vi "Initialize Engine.vi"(8 "error in (no error)":errorcluster, 11 "Abstract Engine":refnum<class "Abstract Engine.lvclass">) -> (0 "error out":errorcluster, 2 "Engine Data":string[](array[string]), 3 "Abstract Engine out":refnum<class "Abstract Engine.lvclass">)   [LabVIEW 2025, in "Abstract Engine.lvlib" / "Abstract Engine.lvclass"]
uses:
  Abstract Engine.lvclass
  Engine configuration/Engine configuration.lvclass
  Abstract Instrument/Abstract Instrument.lvclass
  Abstract Instrument/Channel.ctl
  Engine configuration/Engine configuration.lvclass/Engine configuration.ctl
  Instrument configuration/Instrument configuration.lvclass
  Instrument configuration/Instrument configuration.lvclass/Instrument configuration.ctl
  Engine Cluster.ctl
  Abstract Engine.lvclass/Abstract Engine.ctl
  Instrument configuration/Read Instrument Setting.vi
  Engine configuration/Read Engine Setting.vi
  Write Engine Cluster.vi
  Users/Public/Documents/Sandia National Labs/TSS Plugin/CEF.lvlibp/Node/ReadChildren.vi
  Users/Public/Documents/Sandia National Labs/TSS Plugin/CEF.lvlibp/serializable configuration/CEF_serializable configuration.lvclass
  Users/Public/Documents/Sandia National Labs/TSS Plugin/CEF.lvlibp/Node/CEF_Node.lvclass
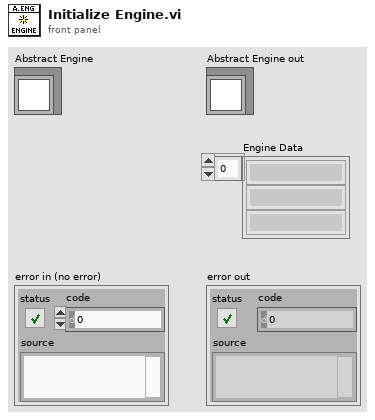
[diagram p1: front panel]
types:
  T1 = typedef "Abstract Engine.lvlib/Abstract Instrument.lvclass/Channel.ctl" = cluster{"Alias":string, "DataType":enum16{"Anaolg Input", "Waveform"}, "Unit":enum16{"---", "V", "A", "Ohm", "Hz", "uF", "degC", "deg"}, "Upper limit":dbl, "Lower limit":dbl, "Measurement":variant}
  T2 = map{string, cluster{"Initialized":bool, "Channels":T1[]}}
  T3 = typedef "Abstract Engine.lvlib/Instrument configuration.lvclass/Default Instrument.ctl" = cluster{"Type":string, "Address":string, "SW Alias":string, "Description":string, "Enabled":bool}
  T4 = typedef "Abstract Engine.lvlib/Engine configuration.lvclass/Engine Setting.ctl" = cluster{"Enabled":bool, "IP Address":string, "Port":i32, "Description":string, "Type":string, "Version":string}
  T5 = typedef "Abstract Engine.lvlib/Abstract Engine.lvclass/Engine Cluster.ctl" = cluster{"IP Address":string, "Type":string, "Initialized":bool, "InstrumentMap":map{string, cluster{"Initialized":bool, "Channels":T1[]}}}
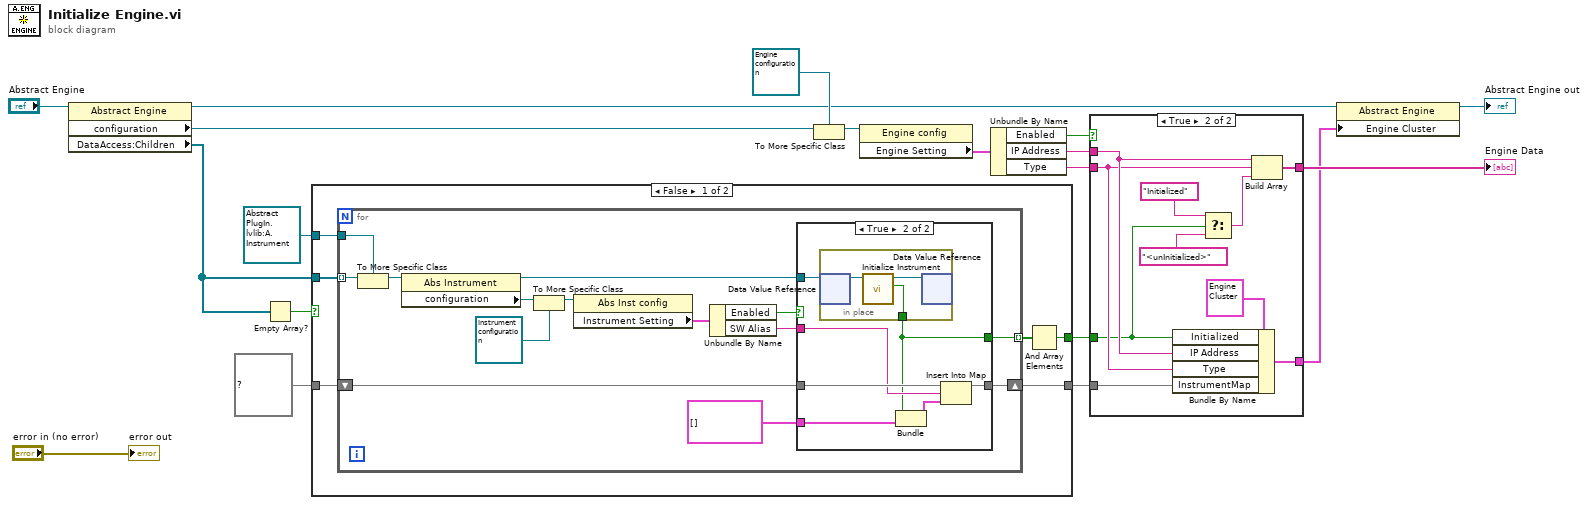
[diagram p0: block diagram]
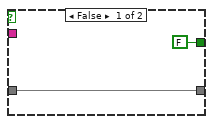
[diagram p2: hidden frame]
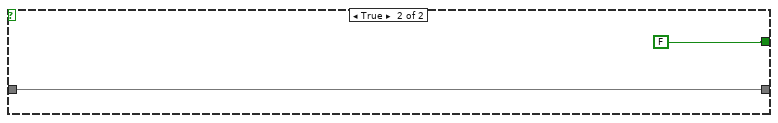
[diagram p3: hidden frame]
diagram:
  n1 = property class="Abstract Engine"(reference="Abstract Engine") -> (reference out=w9:refnum<class "Abstract Engine.lvclass">, "configuration"=w12:refnum<class "CEF_serializable configuration.lvclass">, "DataAccess:Children"=w16:refnum<data-value>[])  [unwired: 1 in, 1 out]
  n2 = Empty Array?(array=w16) -> (empty?=w17:bool)
  n3 = case shown="False" w17 {
    tunnel: [w24 FALSE] -> w4
    tunnel: w16 -> [w23 _]
    tunnel: T2 {} ("InstrumentMap") -> [w22 w52]
    tunnel: [w21 w52] -> w3
    tunnel: refnum<data-value> refnum ("data value reference") -> [w20 _]
    frame False {
      n4 = for {
        tunnel: w23 -> [w38] mode=indexing
        tunnel: [w39] -> w25 mode=indexing
        shift-right: [w30] -> w21
        shift-left: w22 -> [w27]
        tunnel: w20 -> [w28]
        n5 = To More Specific Class(target class=w28, reference=w38) -> (specific class reference=w33:refnum<data-value>)  [unwired: 1 in, 1 out]
        n6 = property class="Abs Instrument"(reference=w33) -> (reference out=w31:refnum<data-value>, "configuration"=w37:refnum<class "CEF_serializable configuration.lvclass">)  [unwired: 1 in, 1 out]
        n7 = To More Specific Class(target class=refnum<class "Instrument configuration.lvclass"> refnum ("Abstract Engine.lvlib:Instrument config"), reference=w37) -> (specific class reference=w35:refnum<class "Instrument configuration.lvclass">)  [unwired: 1 in, 1 out]
        n8 = property class="Abs Inst config"(reference=w35) -> ("Instrument Setting"=w34:T3)  [unwired: 1 in, 2 out]
        n9 = Unbundle By Name(w34) -> ("Enabled"=w29:bool, "SW Alias"=w32:string)
        n10 = case shown="True" w29 {
          tunnel: [FALSE ("Found?") w44] -> w39
          tunnel: w32 -> [_ w45]
          tunnel: w31 -> [_ w48]
          tunnel: w27 -> [w41 w46]
          tunnel: [w41 w47] -> w30
          tunnel: T1[] [] ("Channels") -> [_ w42]
          frame False {
          }
          frame True {
            n11 = in-place {
              in-place-border: [w49] -> w44
              n12 = in-place-dvr #1(w48) -> (w51:refnum<class "Abstract Instrument.lvclass">)  [unwired: 1 out]
              n13 = call "Initialize Instrument.vi"("Abstract Instrument"=w51) -> ("Found?"=w49:bool, "Abstract Instrument out"=w50:refnum<class "Abstract Instrument.lvclass">)  [unwired: 8 in, 1 out]
              n14 = in-place-dvr #1(w50) -> ()  [unwired: 2 out]
            }
            n15 = Bundle("Found?"=w44, "Channels"=w42) -> (w43:cluster{"Found?":bool, "Channels":T1[]})  [unwired: 1 in]
            n16 = Insert Into Map(map in=w46, key=w45, value=w43) -> (map out=w47:T2)  [unwired: 2 out]
          }
        }
      }
      n17 = And Array Elements(Boolean array=w25) -> (logical AND=w24:bool)
    }
    frame True {
    }
  }
  n18 = To More Specific Class(target class=refnum<class "Engine configuration.lvclass"> refnum ("Abstract Engine.lvlib:Engine config"), reference=w12) -> (specific class reference=w13:refnum<class "Engine configuration.lvclass">)  [unwired: 1 in, 1 out]
  n19 = property class="Engine config"(reference=w13) -> ("Engine Setting"=w14:T4)  [unwired: 1 in, 2 out]
  n20 = Unbundle By Name(w14) -> ("Enabled"=w8:bool, "IP Address"=w11:string, "Type"=w7:string)
  n21 = case shown="True" w8 {
    tunnel: [_ w63] -> w5
    tunnel: w11 -> [_ w60]
    tunnel: w7 -> [_ w59]
    tunnel: [_ w62] -> w6
    tunnel: w4 -> [_ w54]
    tunnel: w3 -> [_ w58]
    frame False {
    }
    frame True {
      n22 = Bundle By Name(cluster=T5 {"IP Address"="", "Type"="", "Initialized"=FALSE, "InstrumentMap"={}} ("Engine Cluster"), "Initialized"=w54, "IP Address"=w60, "Type"=w59, "InstrumentMap"=w58) -> (w63:T5)
      n23 = Select(t="Initialized" ("Alias"), s=w54, f="<unInitialized>" ("Alias")) -> (s? t:f=w55:string)
      n24 = Build Array(w60, w59, w55) -> (w62:string[])
    }
  }
  "Engine Data" <- w6
  n25 = property class="Abstract Engine"(reference=w9, "Engine Cluster"=w5) -> (reference out=→"Abstract Engine out":refnum<class "Abstract Engine.lvclass">)  [unwired: 1 in, 1 out]
  "error out" <- "error in (no error)"
